vi "Close_main_SubVI.vi"(1 "output cluster":T26 {"A/SPI - LiDAR"."SPI Configuration"."Frame Length" min=1 max=16}) -> (0 "error constant":errorcluster)   [LabVIEW 2018]
uses:
  <vilib>/myRIO/Instrument Drivers/Onboard IO/DIO/typedefs/DIO Reference.ctl
  <vilib>/myRIO/Common/Instrument Driver Framework/Utilities/typedefs/myRIO Generic Hardware Reference.ctl
  <vilib>/myRIO/Common/Instrument Driver Framework/Utilities/typedefs/Hardware Version Enum.ctl
  <vilib>/myRIO/Common/Instrument Driver Framework/Utilities/typedefs/myRIO v1.0 Reference.ctl
  <vilib>/myRIO/Common/Instrument Driver Framework/Utilities/typedefs/Generic FPGA Reference.ctl
  <vilib>/myRIO/Common/Instrument Driver Framework/myRIO v1.0/DIO/typedefs/DIO Channels List.ctl
  <vilib>/myRIO/Common/Instrument Driver Framework/myRIO v1.0/DIO/typedefs/DIO Channels Enum.ctl
  <vilib>/myRIO/Instrument Drivers/Onboard IO/PWM/typedefs/PWM Reference.ctl
  <vilib>/myRIO/Common/Instrument Driver Framework/myRIO v1.0/PWM/typedefs/PWM Channels Enum.ctl
  <vilib>/myRIO/Instrument Drivers/Onboard IO/PWM/typedefs/PWM Configuration.ctl
  <vilib>/myRIO/Instrument Drivers/Onboard Devices/Accelerometer/typedefs/Accelerometer Reference.ctl
  <vilib>/myRIO/Common/Instrument Driver Framework/myRIO v1.0/Accelerometer/typedefs/Accelerometer Channels List.ctl
  <vilib>/myRIO/Common/Instrument Driver Framework/myRIO v1.0/Accelerometer/typedefs/Accelerometer Channels Enum.ctl
  <vilib>/myRIO/Instrument Drivers/Onboard IO/AI/typedefs/AI Reference.ctl
  <vilib>/myRIO/Common/Instrument Driver Framework/myRIO v1.0/AI/typedefs/AI Channels List.ctl
  <vilib>/myRIO/Common/Instrument Driver Framework/myRIO v1.0/AI/typedefs/AI Channels Enum.ctl
  <vilib>/myRIO/Common/Instrument Driver Framework/Utilities/typedefs/Analog Scaling Constants List.ctl
  <vilib>/myRIO/Common/Instrument Driver Framework/Utilities/typedefs/Analog Scaling Constants.ctl
  <vilib>/myRIO/Instrument Drivers/Onboard IO/SPI/typedefs/SPI Reference.ctl
  <vilib>/myRIO/Common/Instrument Driver Framework/myRIO v1.0/SPI/typedefs/SPI Channels Enum.ctl
  <vilib>/myRIO/Instrument Drivers/Onboard IO/SPI/typedefs/SPI Configuration.ctl
  <vilib>/myRIO/Common/Instrument Driver Framework/myRIO v1.0/SPI/typedefs/SPI Clock Phase.ctl
  <vilib>/myRIO/Common/Instrument Driver Framework/myRIO v1.0/SPI/typedefs/SPI Clock Polarity.ctl
  <vilib>/myRIO/Common/Instrument Driver Framework/myRIO v1.0/SPI/typedefs/SPI Data Direction.ctl
  <vilib>/myRIO/Common/Instrument Driver Framework/myRIO v1.0/SPI/typedefs/SPI Frame Length.ctl
  <vilib>/myRIO/Common/Instrument Driver Framework/myRIO v1.0/DIO/vis/myRIO v1.0 Close DIO.vi
  <vilib>/myRIO/Common/Instrument Driver Framework/myRIO v1.0/SPI/vis/myRIO v1.0 Close SPI.vi
  <vilib>/myRIO/Common/Instrument Driver Framework/myRIO v1.0/AI/vis/myRIO v1.0 Close AI.vi
  <vilib>/myRIO/Common/Instrument Driver Framework/myRIO v1.0/Accelerometer/vis/myRIO v1.0 Close Accelerometer.vi
  <vilib>/myRIO/Common/Instrument Driver Framework/myRIO v1.0/PWM/vis/myRIO v1.0 Close PWM.vi
  <vilib>/myRIO/Common/Instrument Driver Framework/myRIO v1.0/DIO/vis/myRIO v1.0 Unreserve DIO.vi
  <vilib>/myRIO/Common/Instrument Driver Framework/myRIO v1.0/SPI/vis/myRIO v1.0 Unreserve SPI.vi
  <vilib>/myRIO/Common/Instrument Driver Framework/myRIO v1.0/AI/vis/myRIO v1.0 Unreserve AI.vi
  <vilib>/myRIO/Common/Instrument Driver Framework/myRIO v1.0/Accelerometer/vis/myRIO v1.0 Unreserve Accelerometer.vi
  <vilib>/myRIO/Common/Instrument Driver Framework/myRIO v1.0/PWM/vis/myRIO v1.0 Unreserve PWM.vi
  <vilib>/myRIO/Common/Instrument Driver Framework/myRIO v1.0/DIO/vis/myRIO v1.0 Build MUX Configuration DIO.vi
  <vilib>/myRIO/Common/Instrument Driver Framework/myRIO v1.0/Resource Manager/vis/myRIO v1.0 Unreserve Channel List.vi
  <vilib>/myRIO/Common/Instrument Driver Framework/myRIO v1.0/SPI/vis/myRIO v1.0 Build MUX Configuration SPI.vi
  <vilib>/myRIO/Common/Instrument Driver Framework/myRIO v1.0/AI/vis/myRIO v1.0 Build MUX Configuration AI.vi
  <vilib>/myRIO/Common/Instrument Driver Framework/myRIO v1.0/Accelerometer/vis/myRIO v1.0 Build MUX Configuration Accelerometer.vi
  <vilib>/myRIO/Common/Instrument Driver Framework/myRIO v1.0/PWM/vis/myRIO v1.0 Build MUX Configuration PWM.vi
  <vilib>/myRIO/Common/Instrument Driver Framework/myRIO v1.0/Resource Manager/vis/myRIO v1.0 Create Configuration List.vi
  <vilib>/myRIO/Common/Instrument Driver Framework/myRIO v1.0/Resource Manager/vis/myRIO v1.0 Unreserve Channel.vi
  <vilib>/myRIO/Common/Instrument Driver Framework/myRIO v1.0/Resource Manager/vis/myRIO v1.0 Build Mutex Name.vi
  <vilib>/myRIO/Common/Instrument Driver Framework/myRIO v1.0/DIO/vis/myRIO v1.0 Shutdown DIO.vi
  <vilib>/Utility/error.llb/Error Cluster From Error Code.vi
  <vilib>/myRIO/Common/Instrument Driver Framework/myRIO v1.0/Resource Manager/vis/myRIO v1.0 Configure IO.vi
  <vilib>/myRIO/Common/Instrument Driver Framework/Utilities/vis/Configuration Manager.vi
  <vilib>/myRIO/Common/Instrument Driver Framework/Utilities/vis/IO Manager.vi
  <vilib>/myRIO/Common/Instrument Driver Framework/myRIO v1.0/myRIO v1.0 Close.vi
  <vilib>/myRIO/Common/Instrument Driver Framework/myRIO v1.0/SPI/vis/myRIO v1.0 Shutdown SPI.vi
  <vilib>/myRIO/Common/Instrument Driver Framework/myRIO v1.0/PWM/vis/myRIO v1.0 Shutdown PWM.vi
  <vilib>/myRIO/Instrument Drivers/Onboard IO/DIO/DIO.lvlib
  <vilib>/myRIO/Instrument Drivers/Onboard IO/PWM/PWM.lvlib
  <vilib>/myRIO/Instrument Drivers/Onboard IO/AI/AI.lvlib
  <vilib>/myRIO/Instrument Drivers/Onboard Devices/Accelerometer/Accelerometer.lvlib
  <vilib>/myRIO/Instrument Drivers/Onboard IO/SPI/SPI.lvlib
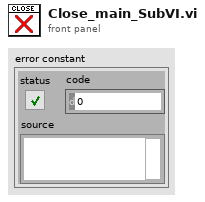
[diagram p1: front panel]
types:
  T1 = typedef "DIO.lvlib/DIO Reference.ctl" = cluster{"myRIO Reference":T2, "DIO Channels List":T6}
  T2 = typedef "myRIO Generic Hardware Reference.ctl" = cluster{"myRIO Model":T3, "myRIO Hardware Reference":T4}
  T3 = typedef "Hardware Version Enum.ctl" = enum16{"Unknown", "myRIO-1900", "myRIO-1950", "roboRIO", "NI ELVIS RIO CM", "ELVIS III"}
  T4 = typedef "myRIO v1.0 Reference.ctl" = cluster{"Generic FPGA Reference":T5, "Allow multiple opens":bool}
  T5 = typedef "Generic FPGA Reference.ctl" = refnum<k20>
  T6 = typedef "DIO Channels List.ctl" = T7[]
  T7 = typedef "DIO Channels Enum.ctl" = enum16{"Not Connected", "C/DIO0", "C/DIO1", "C/DIO2", "C/DIO3", "C/DIO4", "C/DIO5", "C/DIO6", "C/DIO7", "A/DIO0", "A/DIO1", "A/DIO2", "A/DIO3", "A/DIO4", "A/DIO5", "A/DIO6", "A/DIO7", "A/DIO8", "A/DIO9", "A/DIO10", "A/DIO11", "A/DIO12", "A/DIO13", "A/DIO14", "A/DIO15", "A/DIO16", "A/DIO17", "A/DIO18", "A/DIO19", "B/DIO0", "B/DIO1", "B/DIO2", "B/DIO3", "B/DIO4", "B/DIO5", "B/DIO6", "B/DIO7", "B/DIO8", "B/DIO9", "B/DIO10", "B/DIO11", "B/DIO12", "B/DIO13", "B/DIO14", "B/DIO15", "B/DIO16", "B/DIO17", "B/DIO18", "B/DIO19", "LED0", "LED1", "LED2", "LED3", "Button0", "DIO/DIO0", "DIO/DIO1", "DIO/DIO2", "DIO/DIO3", "DIO/DIO4", "DIO/DIO5", "DIO/DIO6", "DIO/DIO7", "DIO/DIO8", "DIO/DIO9", "SPI/CS0", "SPI/CS1", "SPI/CS2", "SPI/CS3", "LED RADIO (Green)", "LED RADIO (Red)", "LED COMM (Green)", "LED COMM (Red)", "LED MODE (Green)", "LED MODE (Red)"}
  T8 = typedef "PWM.lvlib/PWM Reference.ctl" = cluster{"myRIO Reference":T2, "PWM Channels Enum":T9, "PWM Configuration":T10}
  T9 = typedef "PWM Channels Enum.ctl" = enum16{"Not Connected", "C/PWM0", "C/PWM1", "A/PWM0", "A/PWM1", "A/PWM2", "A/PWM3", "A/PWM4", "A/PWM5", "A/PWM6", "A/PWM7", "A/PWM8", "A/PWM9", "A/PWM10", "A/PWM11", "A/PWM12", "A/PWM13", "A/PWM14", "A/PWM15", "A/PWM16", "A/PWM17", "A/PWM18", "A/PWM19", "B/PWM0", "B/PWM1", "B/PWM2", "B/PWM3", "B/PWM4", "B/PWM5", "B/PWM6", "B/PWM7", "B/PWM8", "B/PWM9", "B/PWM10", "B/PWM11", "B/PWM12", "B/PWM13", "B/PWM14", "B/PWM15", "B/PWM16", "B/PWM17", "B/PWM18", "B/PWM19", "PWM/PWM0", "PWM/PWM1", "PWM/PWM2", "PWM/PWM3", "PWM/PWM4", "PWM/PWM5", "PWM/PWM6", "PWM/PWM7", "PWM/PWM8", "PWM/PWM9"}
  T10 = typedef "PWM.lvlib/PWM Configuration.ctl" = cluster{"Frequency":dbl, "Duty Cycle":dbl}
  T11 = typedef "Accelerometer.lvlib/Accelerometer Reference.ctl" = cluster{"myRIO Reference":T2, "Accelerometer Channels List":T12, "LSB Weight":dbl}
  T12 = typedef "Accelerometer Channels List.ctl" = T13[]
  T13 = typedef "Accelerometer Channels Enum.ctl" = enum16{"Not Connected", "X-Axis", "Y-Axis", "Z-Axis"}
  T14 = typedef "AI.lvlib/AI Reference.ctl" = cluster{"myRIO Reference":T2, "AI Channels List":T15, "AI Scaling Constants List":T17}
  T15 = typedef "AI Channels List.ctl" = T16[]
  T16 = typedef "AI Channels Enum.ctl" = enum16{"Not Connected", "AudioIn/Left", "AudioIn/Right", "C/AI0", "C/AI1", "A/AI0", "A/AI1", "A/AI2", "A/AI3", "A/AI4", "A/AI5", "A/AI6", "A/AI7", "B/AI0", "B/AI1", "B/AI2", "B/AI3", "B/AI4", "B/AI5", "B/AI6", "B/AI7", "AI/AI0", "AI/AI1", "AI/AI2", "AI/AI3", "A/AI0 (DIFF)", "A/AI1 (DIFF)", "A/AI2 (DIFF)", "A/AI3 (DIFF)", "B/AI0 (DIFF)", "B/AI1 (DIFF)", "B/AI2 (DIFF)", "B/AI3 (DIFF)"}
  T17 = typedef "Analog Scaling Constants List.ctl" = T18[]
  T18 = typedef "Analog Scaling Constants.ctl" = cluster{"LSB Weight (Volts)":dbl, "Offset (Volts)":dbl, "Signed?":bool}
  T19 = typedef "SPI.lvlib/SPI Reference.ctl" = cluster{"myRIO Reference":T2, "SPI Channels Enum":T20, "SPI Configuration":T21}
  T20 = typedef "SPI Channels Enum.ctl" = enum16{"Not Connected", "A/SPI", "B/SPI", "SPI/SPI"}
  T21 = typedef "SPI.lvlib/SPI Configuration.ctl" = cluster{"Frequency [Hz]":dbl, "Clock Phase":T22, "Clock Polarity":T23, "Data Direction":T24, "Frame Length":T25}
  T22 = typedef "SPI Clock Phase.ctl" = enum8{"Leading", "Trailing"}
  T23 = typedef "SPI Clock Polarity.ctl" = enum8{"Low", "High"}
  T24 = typedef "SPI Data Direction.ctl" = enum8{"Most significant bit first", "Least significant bit first"}
  T25 = typedef "SPI Frame Length.ctl" = u8
  T26 = cluster{"B/DIO0 - Stepper Direction":T1, "B/DIO1 - Stepper1 Enable":T1, "B/DIO2 - Stepper2 Enable":T1, "B/DIO3 - Stepper3 Enable":T1, "B/DIO4 - Endstop Stepper1 Top":T1, "B/DIO11 - Endstop Stepper1 Bund":T1, "B/DIO12 - Endstop Stepper2 Top":T1, "B/DIO13 - Endstop Stepper2 Bund":T1, "B/DIO14 - Endstop Stepper3 Top":T1, "B/DIO15 - Endstop Stepper3 Bund":T1, "A/DIO0 - Cooler":T1, "A/DIO1 - Beacon drop (dio1)":T1, "A/DIO2 - Beacon drop (dio0)":T1, "A/DIO3 - QuickRelease (dio1)":T1, "A/DIO4 - QuickRelease (dio0)":T1, "A/DIO11 - LiDAR SPI CS":T1, "B/PWM0 - Stepper":T8, "B/PWM1 - Drill":T8, "A/PWM0 - Servo_Roll":T8, "A/PWM1 - Servo_Yaw":T8, "Acc. X-axis":T11, "Acc. Y-axis":T11, "B/AI0 - Drone Grounded F3":T14, "B/AI1 - Drone Drill Gear F4":T14, "B/AI2 - Beacon Drop F5":T14, "B/AI3 - Drone Drill Boost F6":T14, "A/AI0 - Drone Stepper F8":T14, "A/AI1 - Beacon Wiper":T14, "A/AI2 - QuickRelease Wiper":T14, "A/AI3 - Drill Current":T14, "A/SPI - LiDAR":T19, "B/UART - XBee":refnum<visa-resource-name>, "A/UART - A3 GPS":refnum<visa-resource-name>, "RIO Flashing LEDs":T1}
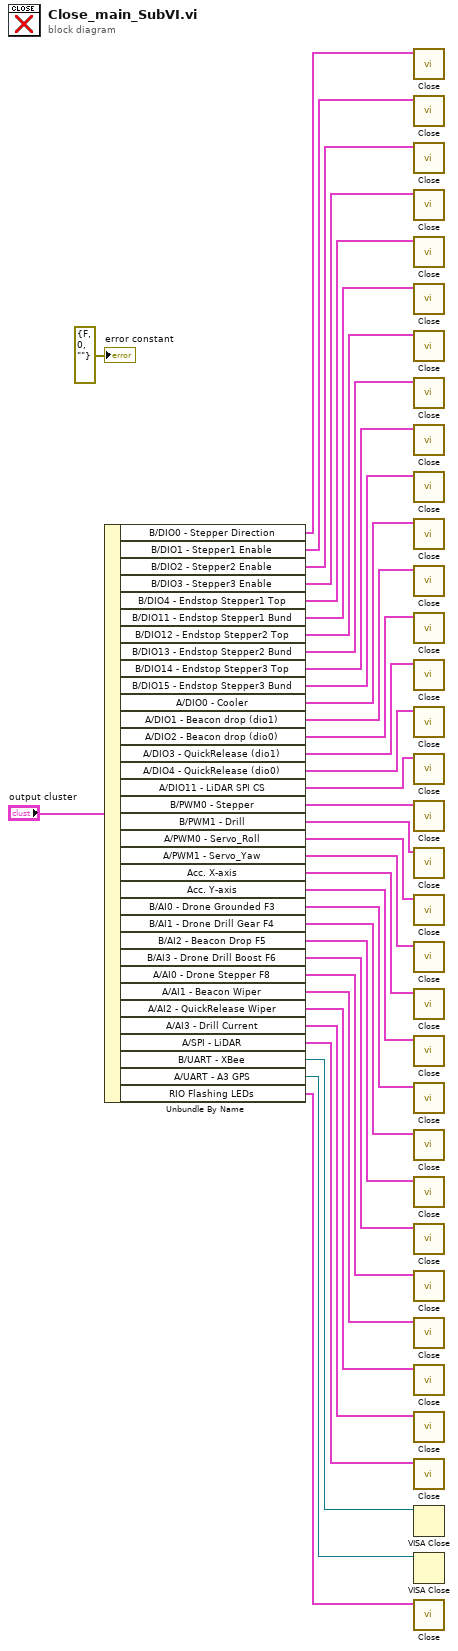
[diagram p0: block diagram]
diagram:
  n1 = Unbundle By Name("output cluster") -> ("B/DIO0 - Stepper Direction"=w20:T1, "B/DIO1 - Stepper1 Enable"=w21:T1, "B/DIO2 - Stepper2 Enable"=w22:T1, "B/DIO3 - Stepper3 Enable"=w23:T1, "B/DIO4 - Endstop Stepper1 Top"=w24:T1, "B/DIO11 - Endstop Stepper1 Bund"=w25:T1, "B/DIO12 - Endstop Stepper2 Top"=w26:T1, "B/DIO13 - Endstop Stepper2 Bund"=w27:T1, "B/DIO14 - Endstop Stepper3 Top"=w28:T1, "B/DIO15 - Endstop Stepper3 Bund"=w29:T1, "A/DIO0 - Cooler"=w30:T1, "A/DIO1 - Beacon drop (dio1)"=w31:T1, "A/DIO2 - Beacon drop (dio0)"=w32:T1, "A/DIO3 - QuickRelease (dio1)"=w33:T1, "A/DIO4 - QuickRelease (dio0)"=w34:T1, "A/DIO11 - LiDAR SPI CS"=w35:T1, "B/PWM0 - Stepper"=w19:T8, "B/PWM1 - Drill"=w16:T8, "A/PWM0 - Servo_Roll"=w17:T8, "A/PWM1 - Servo_Yaw"=w18:T8, "Acc. X-axis"=w4:T11, "Acc. Y-axis"=w3:T11, "B/AI0 - Drone Grounded F3"=w12:T14, "B/AI1 - Drone Drill Gear F4"=w10:T14, "B/AI2 - Beacon Drop F5"=w9:T14, "B/AI3 - Drone Drill Boost F6"=w8:T14, "A/AI0 - Drone Stepper F8"=w7:T14, "A/AI1 - Beacon Wiper"=w6:T14, "A/AI2 - QuickRelease Wiper"=w5:T14, "A/AI3 - Drill Current"=w11:T14, "A/SPI - LiDAR"=w2:T19, "B/UART - XBee"=w14:refnum<visa-resource-name>, "A/UART - A3 GPS"=w15:refnum<visa-resource-name>, "RIO Flashing LEDs"=w13:T1)
  n2 = call <vilib>:"Close.vi"("DIO Ref In"=w20) -> ()  [unwired: 10 in, 1 out]
  n3 = call <vilib>:"Close.vi"("DIO Ref In"=w21) -> ()  [unwired: 10 in, 1 out]
  n4 = call <vilib>:"Close.vi"("DIO Ref In"=w22) -> ()  [unwired: 10 in, 1 out]
  n5 = call <vilib>:"Close.vi"("DIO Ref In"=w23) -> ()  [unwired: 10 in, 1 out]
  n6 = call <vilib>:"Close.vi"("DIO Ref In"=w24) -> ()  [unwired: 10 in, 1 out]
  n7 = call <vilib>:"Close.vi"("DIO Ref In"=w25) -> ()  [unwired: 10 in, 1 out]
  n8 = call <vilib>:"Close.vi"("DIO Ref In"=w26) -> ()  [unwired: 10 in, 1 out]
  n9 = call <vilib>:"Close.vi"("DIO Ref In"=w27) -> ()  [unwired: 10 in, 1 out]
  n10 = call <vilib>:"Close.vi"("DIO Ref In"=w28) -> ()  [unwired: 10 in, 1 out]
  n11 = call <vilib>:"Close.vi"("DIO Ref In"=w29) -> ()  [unwired: 10 in, 1 out]
  n12 = call <vilib>:"Close.vi"("DIO Ref In"=w30) -> ()  [unwired: 10 in, 1 out]
  n13 = call <vilib>:"Close.vi"("DIO Ref In"=w31) -> ()  [unwired: 10 in, 1 out]
  n14 = call <vilib>:"Close.vi"("DIO Ref In"=w32) -> ()  [unwired: 10 in, 1 out]
  n15 = call <vilib>:"Close.vi"("DIO Ref In"=w33) -> ()  [unwired: 10 in, 1 out]
  n16 = call <vilib>:"Close.vi"("DIO Ref In"=w34) -> ()  [unwired: 10 in, 1 out]
  n17 = call <vilib>:"Close.vi"("DIO Ref In"=w35) -> ()  [unwired: 10 in, 1 out]
  n18 = call <vilib>:"Close.vi"("PWM Ref In"=w19) -> ()  [unwired: 10 in, 1 out]
  n19 = call <vilib>:"Close.vi"("PWM Ref In"=w16) -> ()  [unwired: 10 in, 1 out]
  n20 = call <vilib>:"Close.vi"("PWM Ref In"=w17) -> ()  [unwired: 10 in, 1 out]
  n21 = call <vilib>:"Close.vi"("PWM Ref In"=w18) -> ()  [unwired: 10 in, 1 out]
  n22 = call <vilib>:"Close.vi"("Accelerometer Ref In"=w4) -> ()  [unwired: 10 in, 1 out]
  n23 = call <vilib>:"Close.vi"("Accelerometer Ref In"=w3) -> ()  [unwired: 10 in, 1 out]
  n24 = call <vilib>:"Close.vi"("AI Ref In"=w12) -> ()  [unwired: 10 in, 1 out]
  n25 = call <vilib>:"Close.vi"("AI Ref In"=w10) -> ()  [unwired: 10 in, 1 out]
  n26 = call <vilib>:"Close.vi"("AI Ref In"=w9) -> ()  [unwired: 10 in, 1 out]
  n27 = call <vilib>:"Close.vi"("AI Ref In"=w8) -> ()  [unwired: 10 in, 1 out]
  n28 = call <vilib>:"Close.vi"("AI Ref In"=w7) -> ()  [unwired: 10 in, 1 out]
  n29 = call <vilib>:"Close.vi"("AI Ref In"=w6) -> ()  [unwired: 10 in, 1 out]
  n30 = call <vilib>:"Close.vi"("AI Ref In"=w5) -> ()  [unwired: 10 in, 1 out]
  n31 = call <vilib>:"Close.vi"("AI Ref In"=w11) -> ()  [unwired: 10 in, 1 out]
  n32 = call <vilib>:"Close.vi"("SPI Ref In"=w2) -> ()  [unwired: 10 in, 1 out]
  n33 = VISA Close(VISA resource name=w14) -> ()  [unwired: 1 in, 1 out]
  n34 = VISA Close(VISA resource name=w15) -> ()  [unwired: 1 in, 1 out]
  n35 = call <vilib>:"Close.vi"("DIO Ref In"=w13) -> ()  [unwired: 10 in, 1 out]
  "error constant" <- errorcluster {"status"=FALSE, "code"=0, "source"=""} ("error constant")
